vi "project.vi"() -> ()   [LabVIEW 2020]
uses:
  <vilib>/LabVIEW Interface for Arduino/LabVIEW Interface for Arduino.lvlib
panel:
  in  "Units (C)":enum16{"Celsius", "Fahrenheit", "Kelvin"}(ring)
  out "IR Indicator":bool
  in  "stop":bool
  out "MotionDetected":u8
  in  "Sensor Pin":u8
  out "Thermometer":dbl(slide) scale=0.0..50.0
  in  "Vcc (5 v)":dbl=5.0
  in  "Thermistor AI Pin (0)":u8
  in  "VISA resource":refnum<visa-resource-name>
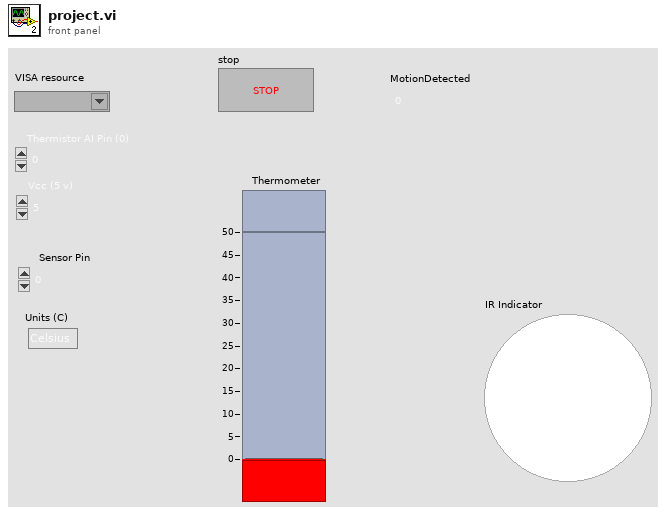
[diagram p1: front panel]
types:
  T1 = typedef "LabVIEW Interface for Arduino.lvlib/Arduino Resource.ctl" = cluster{"VISA resource":refnum<visa-resource-name>, "Board Type":T2, "Connection Type":enum8{"USB / Serial"}, "Bytes Per Packet (15)":u8}
  T2 = typedef "LabVIEW Interface for Arduino.lvlib/Board Type.ctl" = enum16{"Uno", "Dimuelanove w/Atmega 328", "Mega 2560"}
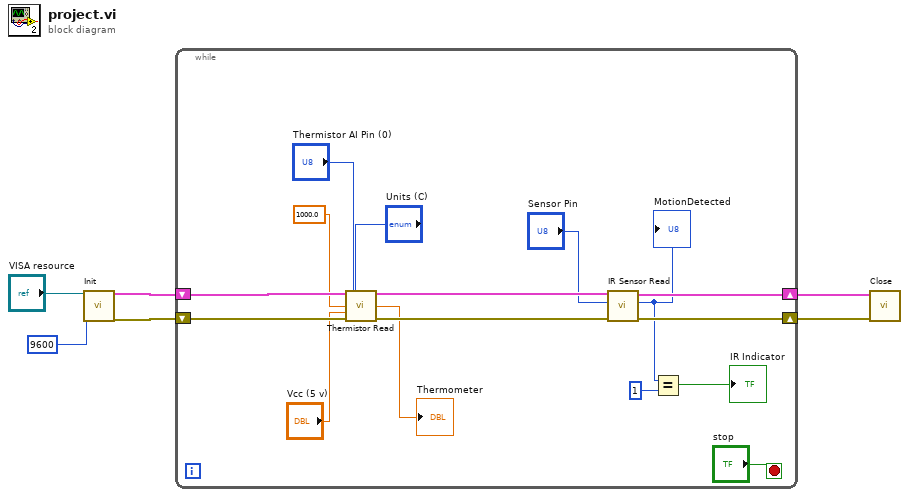
[diagram p0: block diagram]
diagram:
  n1 = call <vilib>:"Init.vi"("VISA resource"="VISA resource", "Baud Rate (115200)"=u32 9600) -> ("Arduino Resource"=w6:T1, "error out"=w5:errorcluster)  [unwired: 16 in]
  n2 = while {
    shift-right: [w18] -> w4
    shift-left: w6 -> [w22]
    shift-right: [w17] -> w3
    shift-left: w5 -> [w21]
    stop <- "stop" stop-if-true
    n3 = call <vilib>:"Thermistor Read.vi"("Arduino Resource"=w22, "Units (C)"="Units (C)", "Thermistor AI Pin (0)"="Thermistor AI Pin (0)", "Paired Resistance (10K Ohms)"=1000.0, "Vcc (5 v)"="Vcc (5 v)", "error in"=w21) -> ("Arduino Resource"=w20:T1, "Temperature"=→"Thermometer":dbl, "error out"=w19:errorcluster)  [unwired: 7 in]
    n4 = call <vilib>:"IR Sensor Read.vi"("error in"=w19, "Sensor Pin"="Sensor Pin", "Arduino Resource"=w20) -> ("error out"=w17:errorcluster, "MotionDetected"=w9:u8, "Arduino Resource"=w18:T1)  [unwired: 6 in]
    "MotionDetected" <- w9
    n5 = Equal?(x=w9, y=u8 1) -> (x = y?=→"IR Indicator":bool)
  }
  n6 = call <vilib>:"Close.vi"("Arduino Resource"=w4, "error in"=w3) -> ()  [unwired: 13 in, 1 out]
